vi "ExtractDeviceInfo.vi"(0 "Line IN":string) -> (1 "valid record?":bool, 2 "Device Info":T1={"Sensor Serial No.:"="", "Wafer:"="", "Batch:"="", "Manufacturer:"="Hamamatsu", "Device Category:"="ATLAS18SS", "Database Serial No.:"="", "Institution"="", "Current Location"="", "Assembled?"=FALSE, "Component:"="SENSOR"})   [LabVIEW 2013]
uses:
  <vilib>/regexp/Match Regular Expression.xnode
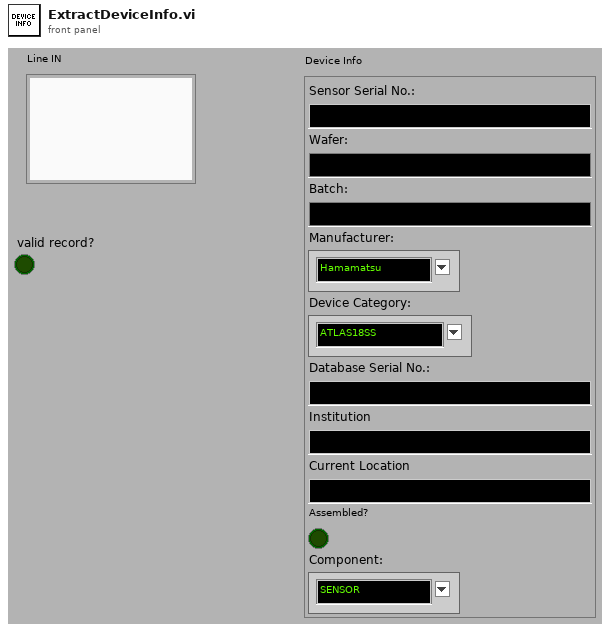
[diagram p1: front panel]
types:
  T1 = cluster{"Sensor Serial No.:":string, "Wafer:":string, "Batch:":string, "Manufacturer:":string, "Device Category:":string, "Database Serial No.:":string, "Institution":string, "Current Location":string, "Assembled?":bool, "Component:":string}
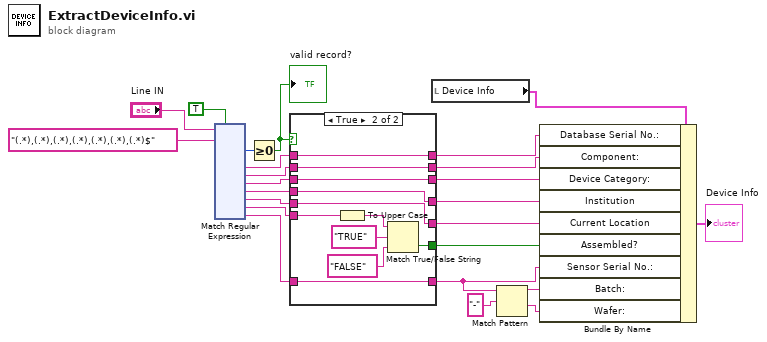
[diagram p0: block diagram]
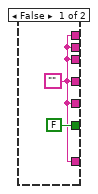
[diagram p2: hidden frame]
diagram:
  n1 = xnode "Match Regular Expression"("input string"="Line IN", "regular expression"="(.*),(.*),(.*),(.*),(.*),(.*),(.*)$", "ignore case? (F)"=TRUE) -> ("offset past match"=w21:i32, "submatch 1"=w19:string, "submatch 2"=w18:string, "submatch 3"=w17:string, "submatch 4"=w16:string, "submatch 5"=w15:string, "submatch 6"=w14:string, "submatch 7"=w2:string)  [unwired: 3 in, 4 out]
  n2 = Greater Or Equal To 0?(x=w21) -> (x >= 0?=w20:bool)
  "valid record?" <- w20
  n3 = case shown="True" w20 {
    tunnel: w19 -> [_ w37]
    tunnel: [w25 w37] -> w7
    tunnel: w18 -> [_ w36]
    tunnel: [w25 w36] -> w6
    tunnel: w17 -> [_ w35]
    tunnel: [w25 w35] -> w5
    tunnel: w16 -> [_ w34]
    tunnel: [w25 w34] -> w4
    tunnel: w15 -> [_ w33]
    tunnel: [w25 w33] -> w3
    tunnel: w14 -> [_ w32]
    tunnel: [FALSE ("selection") w28] -> w11
    tunnel: w2 -> [_ w27]
    tunnel: [w25 w27] -> w1
    frame False {
      w25 = ""
    }
    frame True {
      n4 = To Upper Case(1:w32) -> (0:w31:string)
      n5 = Match True/False String(2:"FALSE" ("false string"), 3:"TRUE" ("true string"), 4:w31) -> (0:w28:bool)  [unwired: 1 out]
    }
  }
  n6 = local read "Device Info"() -> (w12:T1)
  n7 = Match Pattern(string=w1, regular expression="-") -> (before substring=w9:string, after substring=w8:string)  [unwired: 1 in, 2 out]
  n8 = Bundle By Name(cluster=w12, "Database Serial No.:"=w7, "Component:"=w6, "Device Category:"=w5, "Institution"=w4, "Current Location"=w3, "Assembled?"=w11, "Sensor Serial No.:"=w1, "Batch:"=w9, "Wafer:"=w8) -> (→"Device Info":T1)
